vi "Database Connnection Delete Data.vi"(8 "error in (no error)":errorcluster caption="错误输入（无错误）", 9 "condition":string, 10 "table":string, 11 "Database Connection 输入":refnum<class "Database Connection.lvclass"> caption="DNL_LabVIEW Object in") -> (0 "error out":errorcluster caption="错误输出", 3 "Database Connection 输出":refnum<class "Database Connection.lvclass"> caption="DNL_LabVIEW Object out")   [LabVIEW 2011, in "Database Connection.lvclass"]
uses:
  Database Connection.lvclass
  Recordset/Database Recordset.lvclass
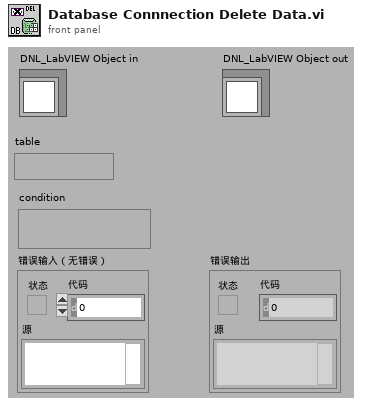
[diagram p1: front panel]
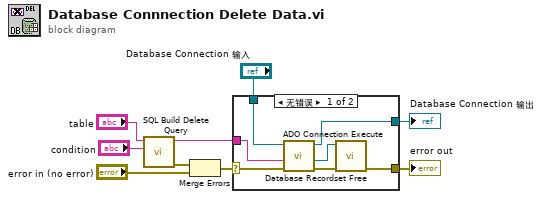
[diagram p0: block diagram]
diagram:
  n1 = call "SQL Build Delete Query.vi"("condition"="condition", "table"="table") -> ("error out"=w4:errorcluster, "Delect"=w1:string)  [unwired: 8 in]
  n2 = Merge Errors(w4, "error in (no error)") -> (w2:errorcluster)
  n3 = case shown="无错误" w2 {
    selector: w2 -> [w13 w18]
    tunnel: [w12 w18] -> w9
    tunnel: [w15 w17] -> w7
    tunnel: "Database Connection 输入" -> [w16 w17]
    tunnel: w1 -> [w10 _]
    frame No Error {
      n4 = call "ADO Connection Execute.vi"("error in (no error)"=w13, "CommandText"=w10, "Database Connection 输入"=w16) -> ("error out"=w11:errorcluster, "Database Recordset输出"=w14:refnum<class "Database Recordset.lvclass">, "Database Connection 输出"=w15:refnum<class "Database Connection.lvclass">)  [unwired: 6 in]
      n5 = call "Database Recordset Free.vi"("error in (no error)"=w11, "Database Recordset 输入"=w14) -> ("error out"=w12:errorcluster)  [unwired: 9 in]
    }
    frame Error {
    }
  }
  "error out" <- w9
  "Database Connection 输出" <- w7
